vi "fmt_escapeXML.vi"(8 "error in":errorcluster, 11 "plain text":string) -> (0 "error out":errorcluster, 3 "xml text":string)   [LabVIEW 2020, in "NI_ExcelFile.lvlib"]
uses:
  <vilib>/express/express shared/NI_ExcelFile/NI_ExcelFile.lvlib
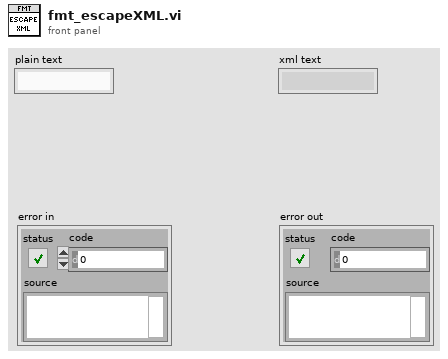
[diagram p1: front panel]
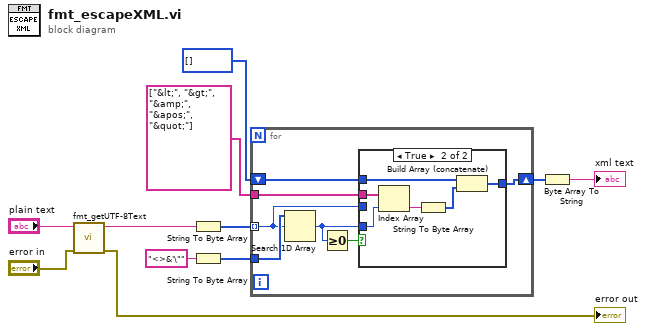
[diagram p0: block diagram]
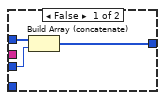
[diagram p2: hidden frame]
diagram:
  n1 = call <vilib>:"fmt_getUTF-8Text.vi"("error in"="error in", "plain text"="plain text") -> ("error out"=→"error out":errorcluster, "utf-8 text"=w1:string)  [unwired: 8 in]
  n2 = String To Byte Array(string=w1) -> (unsigned byte array=w10:u8[])
  n3 = String To Byte Array(string="<>&'\"") -> (unsigned byte array=w9:u8[])
  n4 = for {
    tunnel: w10 -> [w12] mode=indexing
    tunnel: w9 -> [w18]
    tunnel: string[] ["&lt;", "&gt;", "&amp;", "&apos;", "&quot;"] -> [w15]
    shift-right: [w14] -> w7
    shift-left: u8[] [] ("unsigned byte array") -> [w13]
    n5 = Search 1D Array(1D array=w18, element=w12) -> (index of element=w16:i32)  [unwired: 1 in]
    n6 = Greater Or Equal To 0?(x=w16) -> (x >= 0?=w17:bool)
    n7 = case shown="True" w17 {
      tunnel: w16 -> [_ w26]
      tunnel: w15 -> [_ w27]
      tunnel: [w20 w23] -> w14
      tunnel: w13 -> [w21 w22]
      tunnel: w12 -> [w19 _]
      frame False {
        n8 = Build Array (concatenate)(w21, w19) -> (w20:u8[])
      }
      frame True {
        n9 = Index Array(array=w27, index=w26) -> (element=w25:string)
        n10 = String To Byte Array(string=w25) -> (unsigned byte array=w24:u8[])
        n11 = Build Array (concatenate)(w22, w24) -> (w23:u8[])
      }
    }
  }
  n12 = Byte Array To String(unsigned byte array=w7) -> (string=→"xml text":string)
